vi "Vending Machine.vi"() -> ()   [LabVIEW 2020]
uses:
  State of vending machine.ctl
panel:
  in  "Soda with syrup(3 kopeyks)":bool
  in  "Soda without syrup(1 kopeyk)":bool
  out "Total Money":dbl
  in  "Slot":cluster{"1":bool, "2":bool, "3":bool}
  out "Glass":dbl(slide) scale=0.0..10.0
  in  "stop":bool
  out "Ready":bool
  out "Process":string
  out "State":T1
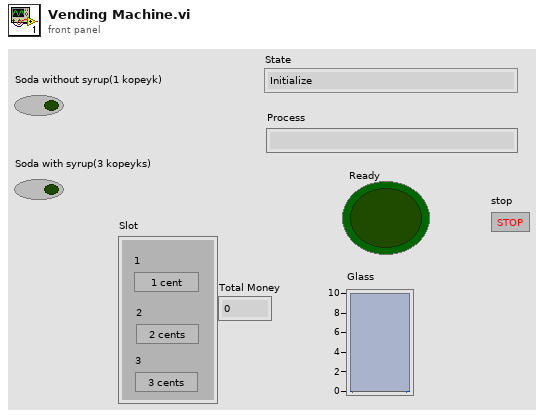
[diagram p1: front panel]
types:
  T1 = typedef "State of vending machine.ctl" = enum16{"Initialize", "Idle", "Busy (without syrup)", "Busy (with syrup)", "Stop", "Add money"}
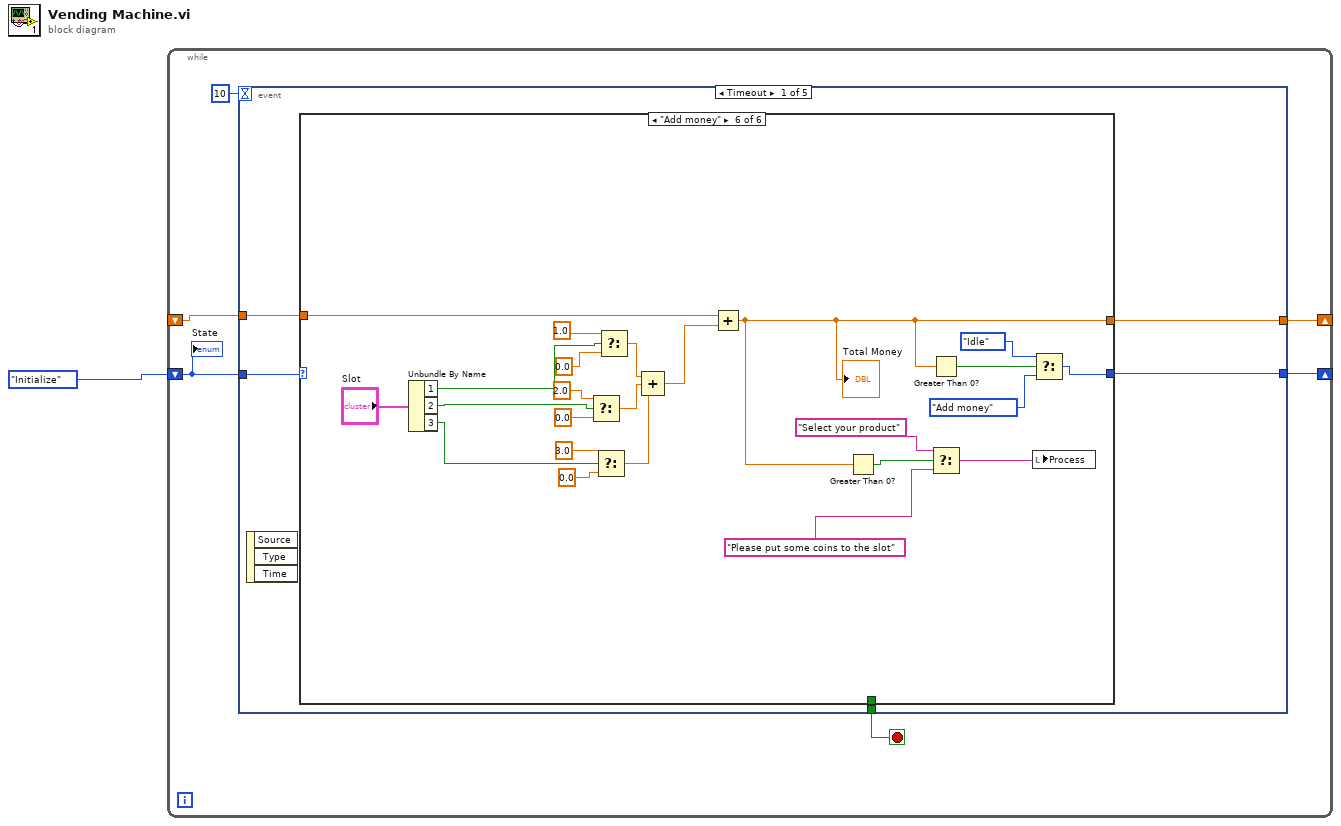
[diagram p0: block diagram]
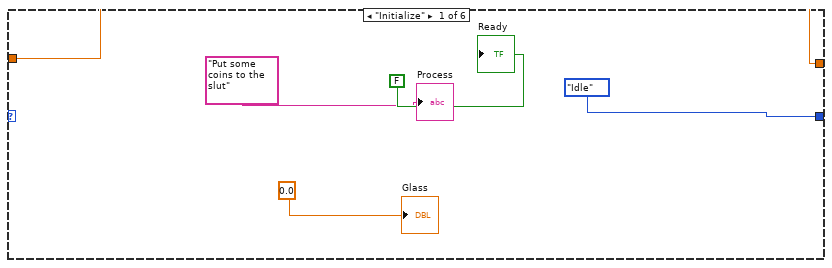
[diagram p2: hidden frame]
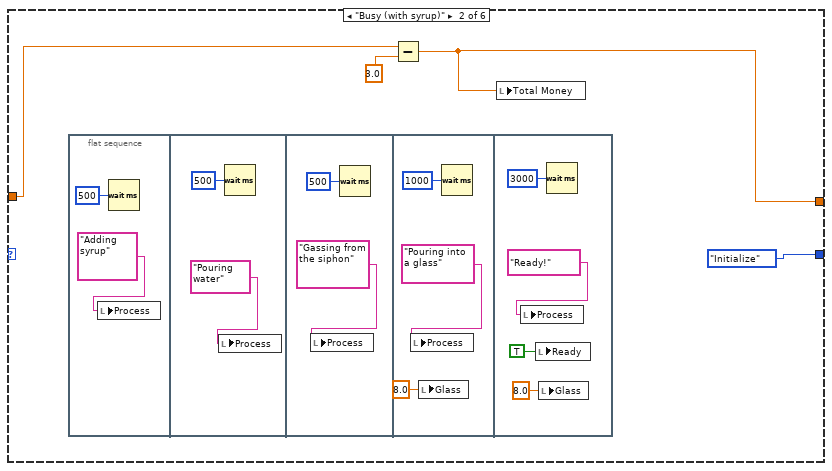
[diagram p3: hidden frame]
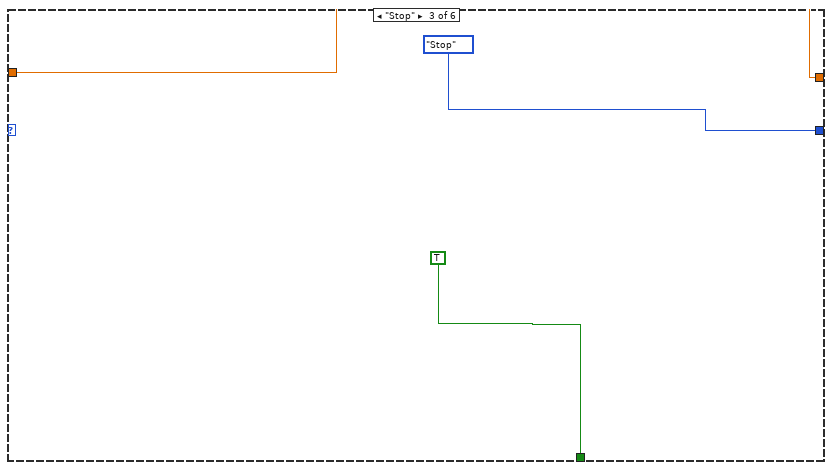
[diagram p4: hidden frame]
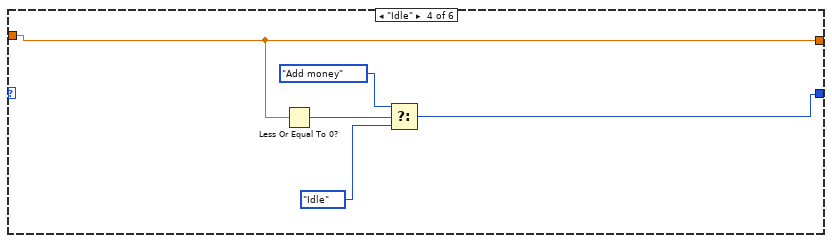
[diagram p5: hidden frame]
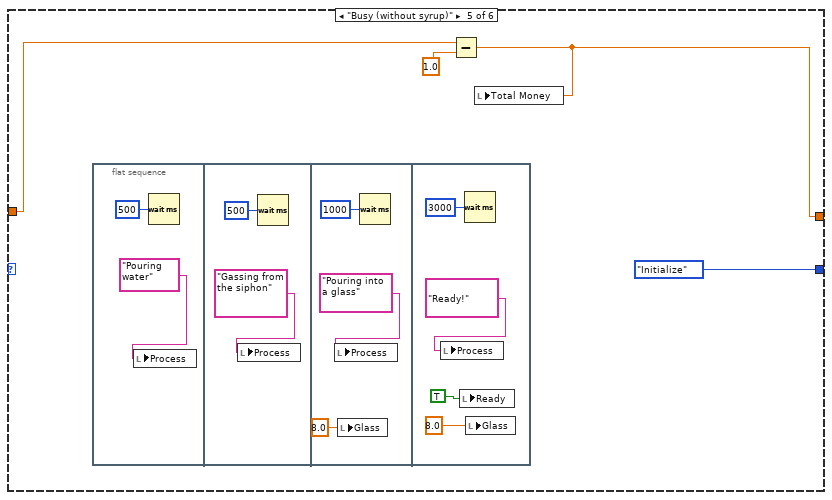
[diagram p6: hidden frame]
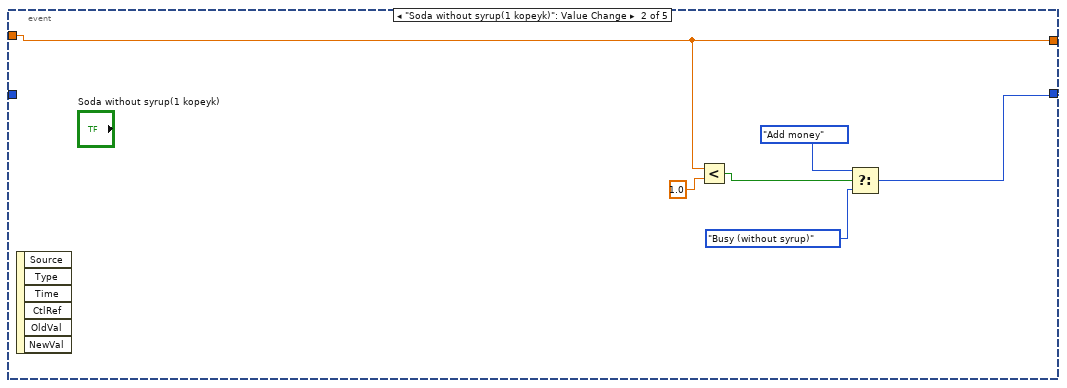
[diagram p7: hidden frame]
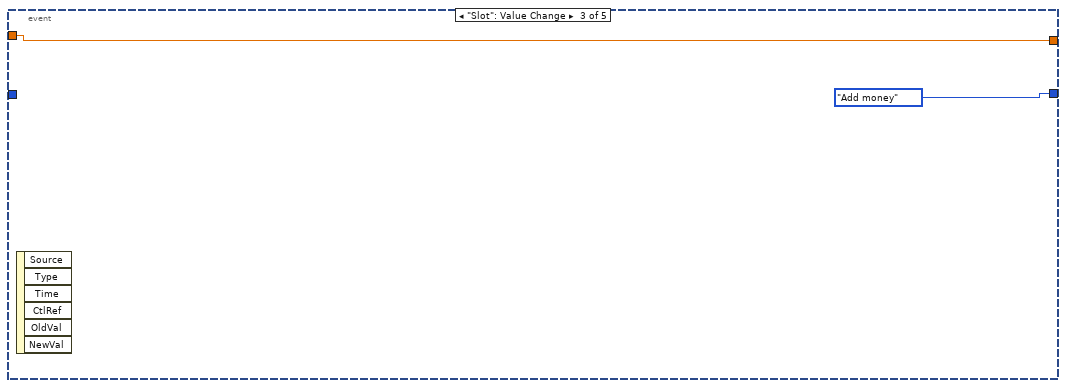
[diagram p8: hidden frame]
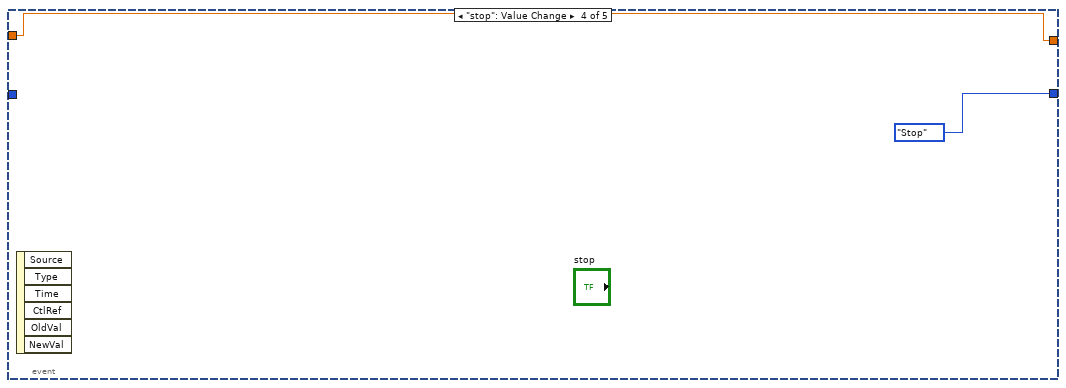
[diagram p9: hidden frame]
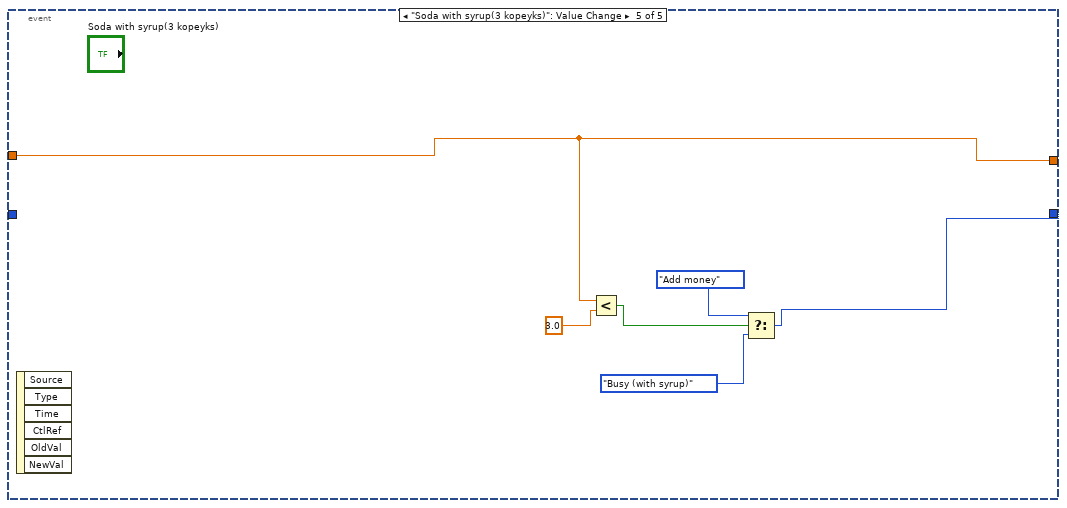
[diagram p10: hidden frame]
diagram:
  n1 = while {
    shift-right: [w7] -> _
    shift-left: State_of_vending_machine."Initialize" -> [w6]
    shift-right: [w2] -> _
    shift-left: _ -> [w4]
    stop <- w5 stop-if-true
    n2 = event shown="[0] Timeout" {
      selector: _ -> [_ _ _ _ _]
      dyn-events: _ -> [_ _ _ _ _]
      timeout: 10 -> [_ _ _ _ _]
      tunnel: [w11 w85 State_of_vending_machine."Add money" State_of_vending_machine."Stop" w96] -> w7
      tunnel: w6 -> [w12 _ _ _ _]
      tunnel: [w10 _ _ _ _] -> w5
      tunnel: w4 -> [w9 w83 w88 w90 w94]
      tunnel: [w8 w83 w88 w90 w94] -> w2
      event Timeout {
        n3 = event-data() -> ()  [unwired: 1 in, 3 out]
        n4 = case shown="\"Add money\"" w12 {
          tunnel: [State_of_vending_machine."Idle" State_of_vending_machine."Initialize" State_of_vending_machine."Stop" w40 State_of_vending_machine."Initialize" w63] -> w11
          tunnel: [_ _ TRUE _ _ _] -> w10
          tunnel: [w13 w19 w35 w42 w44 w67] -> w8
          tunnel: w9 -> [w13 w21 w35 w42 w46 w72]
          frame "Initialize" {
            "Process" <- "Put some coins to the slut"
            "Ready" <- FALSE
            "Glass" <- 0.0 ("Tank")
          }
          frame "Busy (with syrup)" {
            n5 = flat-sequence {
              frame #0 {
                n6 = local write "Process"("Adding syrup") -> ()
                n7 = Wait (ms)(milliseconds to wait=u32 500) -> ()  [unwired: 1 out]
              }
              frame #1 {
                n8 = local write "Process"("Pouring water") -> ()
                n9 = Wait (ms)(milliseconds to wait=u32 500) -> ()  [unwired: 1 out]
              }
              frame #2 {
                n10 = local write "Process"("Gassing from the siphon") -> ()
                n11 = Wait (ms)(milliseconds to wait=u32 500) -> ()  [unwired: 1 out]
              }
              frame #3 {
                n12 = local write "Process"("Pouring into a glass") -> ()
                n13 = local write "Glass"(8.0 ("Tank")) -> ()
                n14 = Wait (ms)(milliseconds to wait=u32 1000) -> ()  [unwired: 1 out]
              }
              frame #4 {
                n15 = local write "Process"("Ready!") -> ()
                n16 = local write "Ready"(TRUE) -> ()
                n17 = local write "Glass"(8.0 ("Tank")) -> ()
                n18 = Wait (ms)(milliseconds to wait=u32 3000) -> ()  [unwired: 1 out]
              }
            }
            n19 = Subtract(x=w21, y=3.0) -> (x-y=w19:dbl)
            n20 = local write "Total Money"(w19) -> ()
          }
          frame "Stop" {
          }
          frame "Idle" {
            n21 = Less Or Equal To 0?(x=w42) -> (x <= 0?=w41:bool)
            n22 = Select(t=State_of_vending_machine."Add money", s=w41, f=State_of_vending_machine."Idle") -> (s? t:f=w40:T1)
          }
          frame "Busy (without syrup)" {
            n23 = flat-sequence {
              frame #0 {
                n24 = local write "Process"("Pouring water") -> ()
                n25 = Wait (ms)(milliseconds to wait=u32 500) -> ()  [unwired: 1 out]
              }
              frame #1 {
                n26 = local write "Process"("Gassing from the siphon") -> ()
                n27 = Wait (ms)(milliseconds to wait=u32 500) -> ()  [unwired: 1 out]
              }
              frame #2 {
                n28 = local write "Process"("Pouring into a glass") -> ()
                n29 = local write "Glass"(8.0 ("Glass")) -> ()
                n30 = Wait (ms)(milliseconds to wait=u32 1000) -> ()  [unwired: 1 out]
              }
              frame #3 {
                n31 = local write "Process"("Ready!") -> ()
                n32 = local write "Ready"(TRUE) -> ()
                n33 = Wait (ms)(milliseconds to wait=u32 3000) -> ()  [unwired: 1 out]
                n34 = local write "Glass"(8.0 ("Glass")) -> ()
              }
            }
            n35 = Subtract(x=w46, y=1.0) -> (x-y=w44:dbl)
            n36 = local write "Total Money"(w44) -> ()
          }
          frame "Add money" {
            n37 = Unbundle By Name("Slot") -> ("1"=w60:bool, "2"=w59:bool, "3"=w58:bool)
            n38 = Select(t=2.0 ("f"), s=w59, f=0.0) -> (s? t:f=w75:dbl)
            n39 = Select(t=3.0 ("f"), s=w58, f=0.0) -> (s? t:f=w74:dbl)
            n40 = Select(t=1.0 ("f"), s=w60, f=0.0) -> (s? t:f=w76:dbl)
            n41 = Compound Arithmetic op=ADD(w76, w75, w74) -> (w73:dbl)
            n42 = Add(x=w72, y=w73) -> (x+y=w67:dbl)
            "Total Money" <- w67
            n43 = Greater Than 0?(x=w67) -> (x > 0?=w71:bool)
            n44 = Greater Than 0?(x=w67) -> (x > 0?=w64:bool)
            n45 = Select(t="Select your product", s=w71, f="Please put some coins to the slot") -> (s? t:f=w68:string)
            n46 = local write "Process"(w68) -> ()
            n47 = Select(t=State_of_vending_machine."Idle", s=w64, f=State_of_vending_machine."Add money") -> (s? t:f=w63:T1)
          }
        }
      }
      event "Soda without syrup(1 kopeyk)": Value Change {
        n48 = event-data() -> ()  [unwired: 1 in, 6 out]
        n49 = Less?(x=w83, y=1.0) -> (x < y?=w82:bool)
        n50 = Select(t=State_of_vending_machine."Add money", s=w82, f=State_of_vending_machine."Busy (without syrup)") -> (s? t:f=w85:T1)
      }
      event "Slot": Value Change {
        n51 = event-data() -> ()  [unwired: 1 in, 6 out]
      }
      event "stop": Value Change {
        n52 = event-data() -> ()  [unwired: 1 in, 6 out]
      }
      event "Soda with syrup(3 kopeyks)": Value Change {
        n53 = event-data() -> ()  [unwired: 1 in, 6 out]
        n54 = Less?(x=w94, y=3.0 ("x")) -> (x < y?=w95:bool)
        n55 = Select(t=State_of_vending_machine."Add money", s=w95, f=State_of_vending_machine."Busy (with syrup)") -> (s? t:f=w96:T1)
      }
    }
    "State" <- w6
  }
